vi "gwyscan save gwyddion xyz.vi"(0 "xypos":dbl[](array[numeric]), 1 "xres":i32, 2 "description":i32[](array[numeric]), 5 "zdata":dbl[](array[numeric]), 7 "n":i32, 9 "nchannels":i32, 11 "error in (no error)":errorcluster, 12 "yres":i32, 13 "filename":string) -> (8 "filename out":string, 10 "function return":i32, 15 "error out":errorcluster)   [LabVIEW 2016, in "libgwyscan.lvlib"]
doc: "GWYSCANDLL_API int gwyscan_save_gwyddion_xyz(double *xypos, double *zdata, int n, int xres, int yres, char *filename);\n\nGWYSCANDLL_API GwyscanResult gwyscan_save_gwyddion_xyz(const double *xypos, const double *zdata, int n, int nchannels, int xres, int yres, const char **description, const char *filename);"
uses:
  libgwyscan.lvlib
  libgwyscan.dll
panel:
  out "xypos":dbl[](array[numeric])
  out "zdata":dbl[](array[numeric])
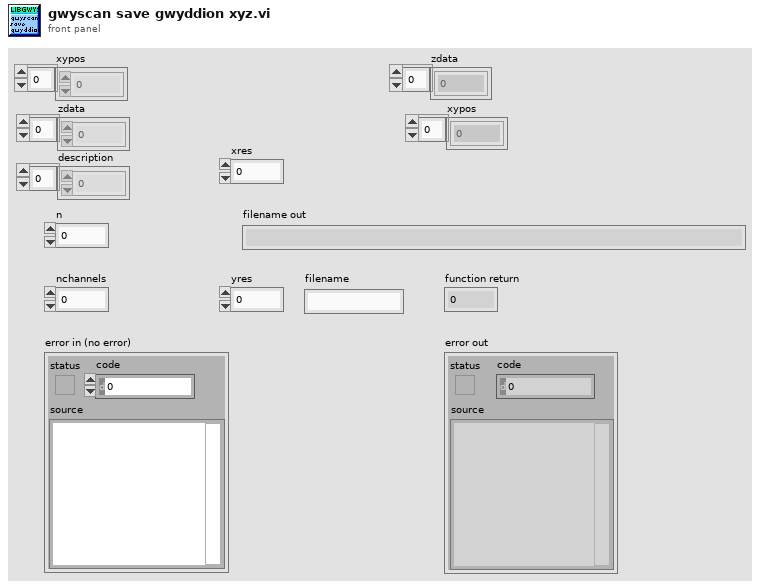
[diagram p1: front panel]
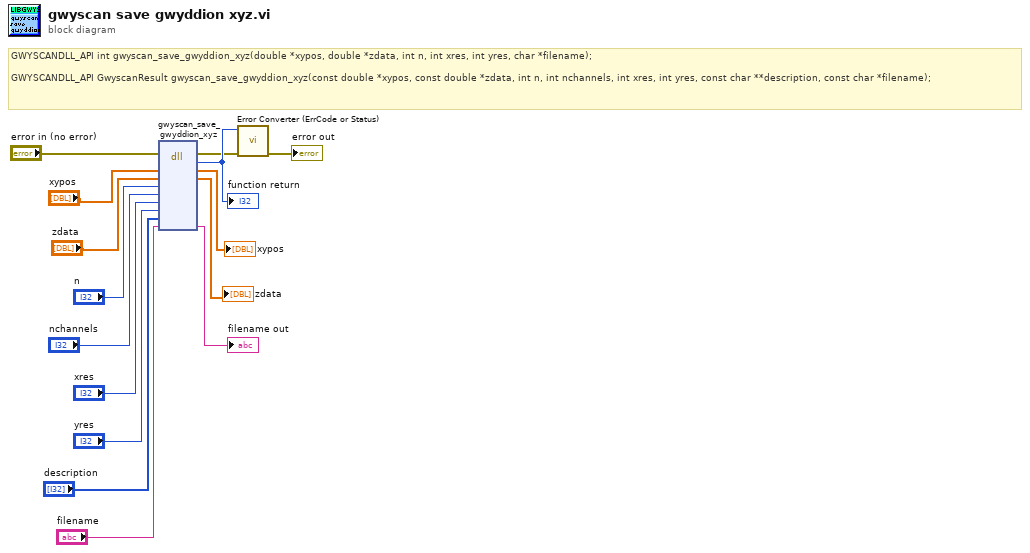
[diagram p0: block diagram]
diagram:
  # "GWYSCANDLL_API int gwyscan_save_gwyddion_xyz(double *xypos, double *zdata, int n, int xres, int yres, char *filename);\n\nGWYSCANDLL_API GwyscanResult gwyscan_save_gwyddion_xyz(const double *xypos, const double *zdata, int n, int nchannels, int xres, int yres, const char **description, const char *filename);"
  n1 = dll-call lib="PTH2abs CUsersCharlÃ¨ne BrillardDesktoplbni-lbniAFMController-BetaVersionv2.0.16-20190611 libgwyscan-1.2-labview2015-win32libgwyscan.*" fn="gwyscan_save_gwyddion_xyz"(error in="error in (no error)", "xypos"="xypos", "zdata"="zdata", "n"="n", "nchannels"="nchannels", "xres"="xres", "yres"="yres", "description"="description", "filename"="filename") -> (error out=w5:errorcluster, "return type"=w15:i32, "xypos"=→"xypos":dbl[], "zdata"=→"zdata":dbl[], "filename"=→"filename out":string)  [unwired: 7 in, 1 out]
  "function return" <- w15
  n2 = call "Error Converter (ErrCode or Status).vi"("error in (no error)"=w5, "error code"=w15) -> ("error out"=→"error out":errorcluster)  [unwired: 9 in]
